vi "Oscilloscope_LongTimeVersion.vi"() -> ()   [LabVIEW 2024]
uses:
  <vilib>/DAQmx/read.llb/DAQmx Read (Analog 1D Wfm NChan NSamp).vi
  <vilib>/DAQmx/create/channels.llb/DAQmx Create Channel (AI-Voltage-Basic).vi
  <vilib>/DAQmx/configure/timing.llb/DAQmx Timing (Sample Clock).vi
  <vilib>/DAQmx/miscellaneous.llb/DAQmx Fill In Error Info.vi
panel:
  in  "y":errorcluster
  out "written":i32
  out "# elementsAfter":i32
  out "# elements Before":i32
  in  "File Duration (seconds per file)":dbl
  in  "File Logging":bool
  in  "TimeRangeMAX (2)":dbl
  in  "AmpRangeMAX (2)":dbl
  in  "AmpRange MAX (1)":dbl
  in  "TimeRangeMAX (1)":dbl
  out "right 2":dynamicdata(graph)=[{"t0"=timestamp(3806599236.6321588 s since 1904-01-01), "dt"=4.999999999999579e-07, "Y"=array[202167 elements], "attributes"=variant("NI_ChannelName"=variant(string "cDAQ2Mod1/ai1"), "NI_UnitDescription"=variant(string "Volts"))}]
  out "left 2":dynamicdata(graph)=[{"t0"=timestamp(3806599236.6321588 s since 1904-01-01), "dt"=4.999999999999579e-07, "Y"=array[202167 elements], "attributes"=variant("NI_ChannelName"=variant(string "cDAQ2Mod1/ai0"), "NI_UnitDescription"=variant(string "Volts"))}]
  in  "stop Acquisition":bool
  in  "Folder to save file to 2":path=path "A:/Source Localization/Material Evaluation paper/Dataset/Microphone Characterization/Clean Source"
  in  "physical channels 2":tag="cDAQ2Mod1/ai0, cDAQ2Mod1/ai3"
  in  "Sample Rate 2":dbl=200000.0 format="%0.2f"
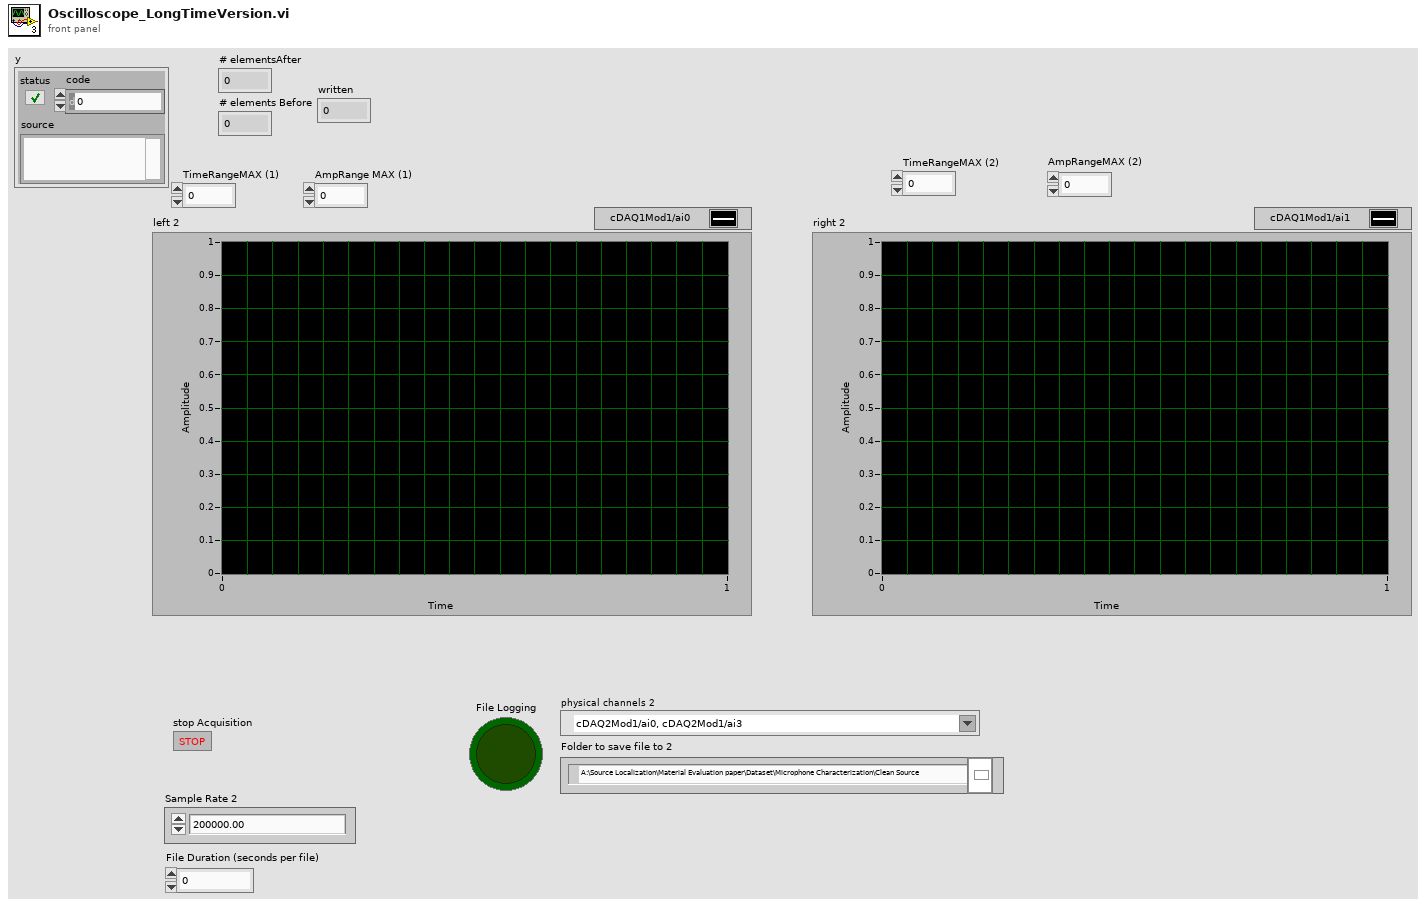
[diagram p1: front panel]
types:
  T1 = enum16{"open", "open or create", "create or replace", "create", "open (read-only)"}
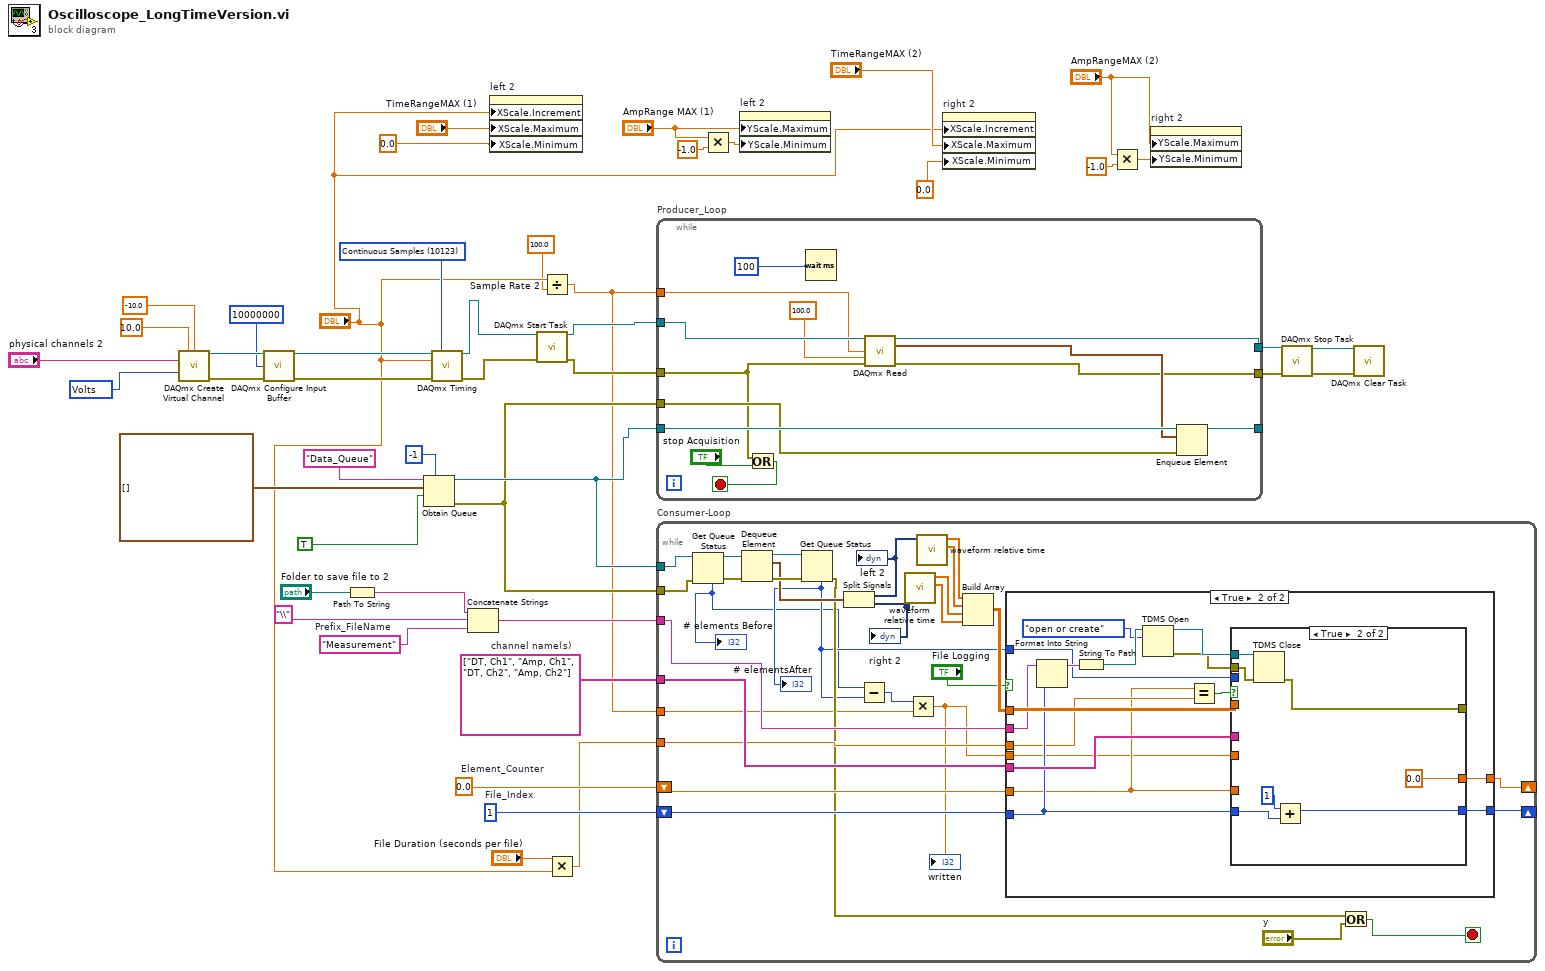
[diagram p0: block diagram]
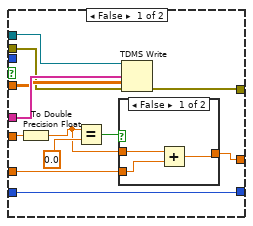
[diagram p3: hidden frame]
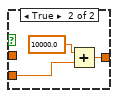
[diagram p4: hidden frame]
diagram:
  w5 = 0.0  # Element_Counter
  w10 = 1  # File_Index
  w9 = "Measurement"  # Prefix_FileName
  w25 = 10348 items=["Volts"=10348, "From Custom Scale"=10065] ("units")
  w27 = string[] ["DT, Ch1", "Amp, Ch1", "DT, Ch2", "Amp, Ch2"]  # channel name(s)
  w42 = 10123 items=["Finite Samples"=10178, "Continuous Samples"=10123, "Hardware Timed Single Point"=12522] ("sample mode")
  n1 = call-poly <vilib>:"DAQmx Create Virtual Channel.vi"("maximum value"=10.0, "minimum value"=-10.0, "physical channels"="physical channels 2", "units"=w25) -> ("task out"=w47:refnum<k21>, "error out"=w46:errorcluster)  [unwired: 10 in]
  n2 = call <vilib>:"DAQmx Configure Input Buffer.vi"("task/channels in"=w47, "buffer size (in samples per channel)"=u32 10000000, "error in"=w46) -> ("task out"=w44:refnum<k21>, "error out"=w43:errorcluster)  [unwired: 11 in]
  n3 = Path To String(path="Folder to save file to 2") -> (string=w37:string)
  n4 = Obtain Queue(max queue size (-1, unlimited)=-1, name (unnamed)="Data_Queue", element data type=waveform(dbl)[] [] ("waveform"), create if not found? (T)=TRUE) -> (queue out=w31:refnum<queue>, error out=w28:errorcluster)  [unwired: 1 in, 1 out]
  n5 = call-poly <vilib>:"DAQmx Timing.vi"("task/channels in"=w44, "sample mode"=w42, "rate"="Sample Rate 2", "error in"=w43) -> ("task out"=w23:refnum<k21>, "error out"=w24:errorcluster)  [unwired: 10 in]
  n6 = Concatenate Strings(w37, "\\" ("string"), w9) -> (w8:string)
  n7 = property on="left 2" class="WFGraph (strict)"("XScale.Increment"="Sample Rate 2", "XScale.Maximum"="TimeRangeMAX (1)", "XScale.Minimum"=0.0 ("X Scale.Range:Minimum")) -> ()  [unwired: 2 in, 2 out]
  n8 = call <vilib>:"DAQmx Start Task.vi"("task/channels in"=w23, "error in"=w24) -> ("task out"=w7:refnum<k21>, "error out"=w6:errorcluster)  [unwired: 12 in]
  n9 = Divide(x="Sample Rate 2", y=100.0) -> (x/y=w1:dbl)
  n10 = Multiply(x="File Duration (seconds per file)", y="Sample Rate 2") -> (x*y=w4:dbl)
  n11 = while "Producer_Loop" {
    tunnel: w7 -> [w59]
    tunnel: w6 -> [w51]
    tunnel: w31 -> [w60]
    tunnel: w28 -> [w52]
    tunnel: [w58] -> _
    tunnel: [w55] -> w30
    tunnel: [w50] -> w29
    tunnel: w1 -> [w48]
    stop <- w56 stop-if-true
    n12 = Or(x=w51, y="stop Acquisition") -> (x .or. y?=w56:bool)
    n13 = Wait (ms)(milliseconds to wait=u32 100) -> ()  [unwired: 1 out]
    n14 = call-poly <vilib>:"DAQmx Read.vi"("task/channels in"=w59, "number of samples per channel"=w48, "timeout"=100.0, "error in"=w51) -> ("task out"=w55:refnum<k21>, "data"=w54:waveform(dbl)[], "error out"=w50:errorcluster)  [unwired: 9 in]
    n15 = Enqueue Element(queue=w60, element=w54, error in (no error)=w52) -> (queue out=w58:refnum<queue>)  [unwired: 1 in, 2 out]
  }
  n16 = while "Consumer-Loop" {
    tunnel: w31 -> [w71]
    tunnel: w28 -> [w70]
    tunnel: w27 -> [w90]
    shift-right: [w67] -> _
    shift-left: w5 -> [w74]
    shift-right: [w78] -> _
    shift-left: w10 -> [w80]
    tunnel: w4 -> [w79]
    tunnel: w8 -> [w77]
    tunnel: w1 -> [w63]
    stop <- w89 stop-if-true
    n17 = Get Queue Status(queue=w71, error in (no error)=w70) -> (queue out=w72:refnum<queue>, error out=w69:errorcluster, # elements in queue=w62:i32)  [unwired: 1 in, 5 out]
    "# elements Before" <- w62
    n18 = Dequeue Element(queue=w72, error in (no error)=w69) -> (queue out=w73:refnum<queue>, element=w75:waveform(dbl)[], error out=w76:errorcluster)  [unwired: 1 in, 1 out]
    n19 = Get Queue Status(queue=w73, error in (no error)=w76) -> (error out=w68:errorcluster, # elements in queue=w66:i32)  [unwired: 1 in, 6 out]
    "# elementsAfter" <- w66
    n20 = Split Signals(w75) -> (w81:dynamicdata, w84:dynamicdata)  [unwired: 2 in]
    "left 2" <- w81
    "right 2" <- w84
    n21 = Subtract(x=w62, y=w66) -> (x-y=w65:i32)
    n22 = call "waveform relative time.vi"("signal in"=w84) -> ("Y"=w88:dbl[], "Relative Time"=w87:dbl[])  [unwired: 7 in, 2 out]
    n23 = Multiply(x=w65, y=w63) -> (x*y=w64:dbl)
    "written" <- w64
    n24 = call "waveform relative time.vi"("signal in"=w81) -> ("Y"=w85:dbl[], "Relative Time"=w86:dbl[])  [unwired: 7 in, 2 out]
    n25 = Build Array(w86, w85, w87, w88) -> (w83:dbl[][])
    n26 = case shown="True" "File Logging" {
      tunnel: w90 -> [_ w107]
      tunnel: w83 -> [_ w106]
      tunnel: w74 -> [w91 w95]
      tunnel: w80 -> [w92 w99]
      tunnel: w79 -> [_ w96]
      tunnel: [w92 w100] -> w78
      tunnel: w77 -> [_ w105]
      tunnel: [w91 w98] -> w67
      tunnel: w66 -> [_ w94]
      tunnel: w64 -> [_ w93]
      frame False {
      }
      frame True {
        n27 = Format Into String(initial string=w105, w99) -> (resulting string=w104:string)  [unwired: 2 in, 1 out]
        n28 = String To Path(string=w104) -> (path=w103:path)
        n29 = TDMS Open(10:T1."open or create" ("operation (0:open)"), 11:w103) -> (0:w97:errorcluster, 3:w101:refnum<k34>)  [unwired: 5 in]
        n30 = Equal?(x=w95, y=w96) -> (x = y?=w108:bool)
        n31 = case shown="True" w108 {
          tunnel: w107 -> [w120 _]
          tunnel: w106 -> [w119 _]
          tunnel: w97 -> [w118 w132]
          tunnel: [w117 w128] -> _
          tunnel: w101 -> [w116 w133]
          tunnel: w95 -> [w114 _]
          tunnel: [w110 0.0] -> w98
          tunnel: w99 -> [w115 w131]
          tunnel: [w115 w129] -> w100
          tunnel: w94 -> [_ _]
          tunnel: w93 -> [w113 _]
          frame False {
            n32 = To Double Precision Float(number=w113) -> (double precision float=w109:dbl)
            n33 = Equal?(x=w109, y=0.0) -> (x = y?=w111:bool)
            n34 = case shown="False" w111 {
              tunnel: w114 -> [w123 w126]
              tunnel: [w121 w124] -> w110
              tunnel: w109 -> [w122 _]
              frame False {
                n35 = Add(x=w122, y=w123) -> (x+y=w121:dbl)
              }
              frame True {
                n36 = Add(x=10000.0, y=w126) -> (x+y=w124:dbl)
              }
            }
            n37 = TDMS Write(0:w116, 7:w120, 9:w119, 11:w118) -> (15:w117:errorcluster)  [unwired: 2 in, 3 out]
          }
          frame True {
            n38 = TDMS Close(8:w132, 11:w133) -> (0:w128:errorcluster)  [unwired: 1 out]
            n39 = Add(x=1, y=w131) -> (x+y=w129:i32)
          }
        }
      }
    }
    n40 = Or(x=w68, y="y") -> (x .or. y?=w89:bool)
  }
  n41 = Multiply(x="AmpRange MAX (1)", y=-1.0) -> (x*y=w19:dbl)
  n42 = property on="left 2" class="WFGraph (strict)"("YScale.Maximum"="AmpRange MAX (1)", "YScale.Minimum"=w19) -> ()  [unwired: 2 in, 2 out]
  n43 = property on="right 2" class="WFGraph (strict)"("XScale.Increment"="Sample Rate 2", "XScale.Maximum"="TimeRangeMAX (2)", "XScale.Minimum"=0.0 ("X Scale.Range:Minimum")) -> ()  [unwired: 2 in, 2 out]
  n44 = Multiply(x="AmpRangeMAX (2)", y=-1.0) -> (x*y=w16:dbl)
  n45 = property on="right 2" class="WFGraph (strict)"("YScale.Maximum"="AmpRangeMAX (2)", "YScale.Minimum"=w16) -> ()  [unwired: 2 in, 2 out]
  n46 = call <vilib>:"DAQmx Stop Task.vi"("task/channels in"=w30, "error in"=w29) -> ("task out"=w36:refnum<k21>, "error out"=w35:errorcluster)  [unwired: 12 in]
  n47 = call <vilib>:"DAQmx Clear Task.vi"("task in"=w36, "error in"=w35) -> ()  [unwired: 13 in, 1 out]
